vi "FindFacesGrabTester_DEPRECATED.vi"() -> ()   [LabVIEW 2017]
uses:
  Camera_IMAQdx_class/Camera_IMAQdx.lvclass
  Camera_IMAQdx_class/typedefs/Configuration--Cluster.ctl
  ImageFacialDetection_class/ImageFacialDetection.lvclass
  <userlib>/_OpenG.lib/comparison/comparison.llb/Boolean Changed__ogtk.vi
  <vilib>/vision/Image Controls.llb/IMAQ Image.ctl
  <vilib>/userdefined/High Color/IMAQdx.ctl
panel:
  in  "Find Faces":bool
  in  "Refresh List":bool
  in  "Snap":bool
  in  "Start Stop Grab":bool
  in  "Connect to Camera":bool
  in  "Cameras":u16(ring) items=["VMware Virtual USB Video Device "]
  out "Image":T1(plugin-control)
  in  "OK":bool
  out "Frame Number:":u32
  out "Connected":bool
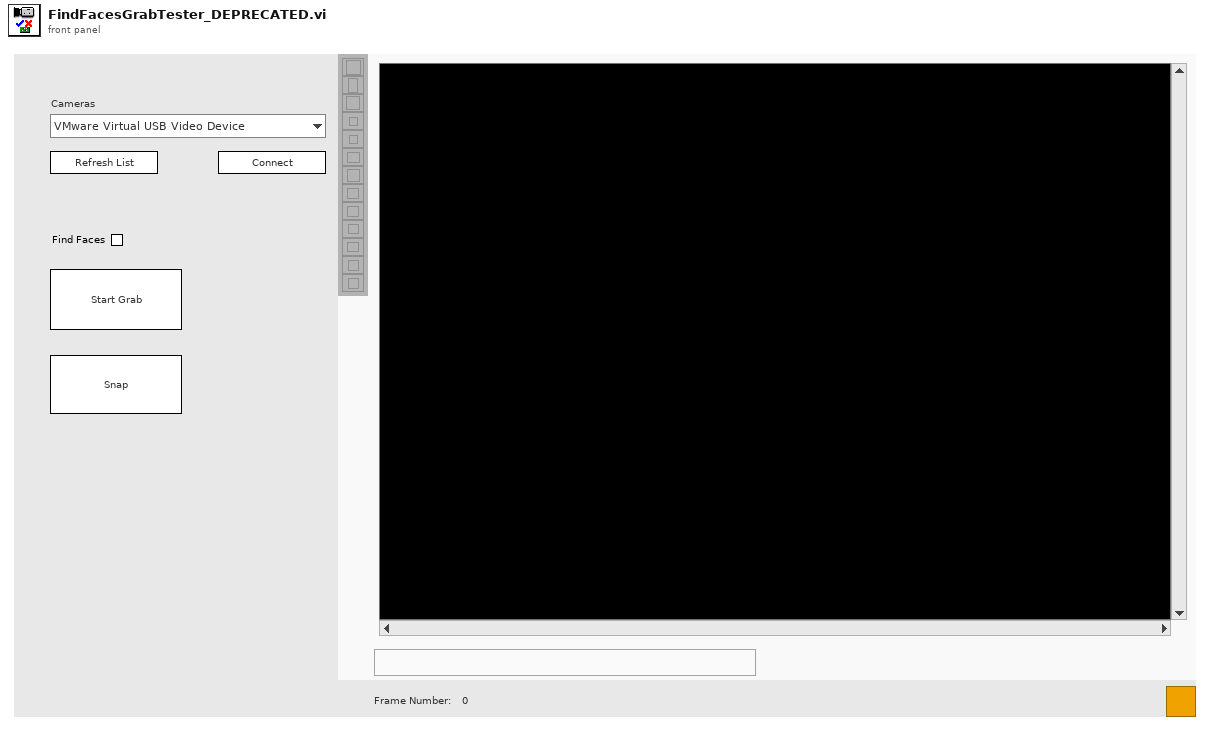
[diagram p1: front panel]
types:
  T1 = typedef "IMAQ Image.ctl" = refnum<image>
  T2 = typedef "Camera_IMAQdx.lvclass/Configuration--Cluster.ctl" = cluster{"Camera Interface Name":string, "Number of Buffers":u32, "Image Name":string, "Image Type":T3}
  T3 = typedef "Image Type" = u32
  T4 = enum32{"invalid app kind", "Development System", "Run Time System", "Student Edition", "Embedded LabVIEW", "Evaluation", "Custom"}
  T5 = enum8{"Enabled", "Disabled", "Disabled and Grayed Out"}
  T6 = enum32{"Invalid", "Standard", "Closed", "Hidden", "Minimized", "Maximized"}
  T7 = cluster{"Core":cluster{"Current VI Reference":refnum<vi>, "Close Panel on Exit?":bool}, "Camera.IMAQdx":refnum<class "Camera_IMAQdx.lvclass">, "All Camera Interfaces":string[], "Connected":bool, "Grabbing":bool, "Find Faces?":bool, "Facial Detection Initialized":bool, "FacialDetection":refnum<class "ImageFacialDetection.lvclass">, "Image":T1, "Face Found":refnum<user-event>, "Frame Complete Event":refnum<event-registration>, "Frame Number":u32}
  T8 = cluster{"Event Registration Refnum":refnum<event-registration>, "Frame Complete Event":refnum<event-registration>}
  T9 = cluster{"Current VI Reference":refnum<vi>, "Close Panel on Exit?":bool}
  T10 = cluster{"Type":u32, "Version":u32, "Flags":u32, "SerialNumberHigh":u32, "SerialNumberLow":u32, "BusType":u32, "InterfaceName":string, "VendorName":string, "ModelName":string, "CameraFileName":string, "CameraAttributeURL":string}[]
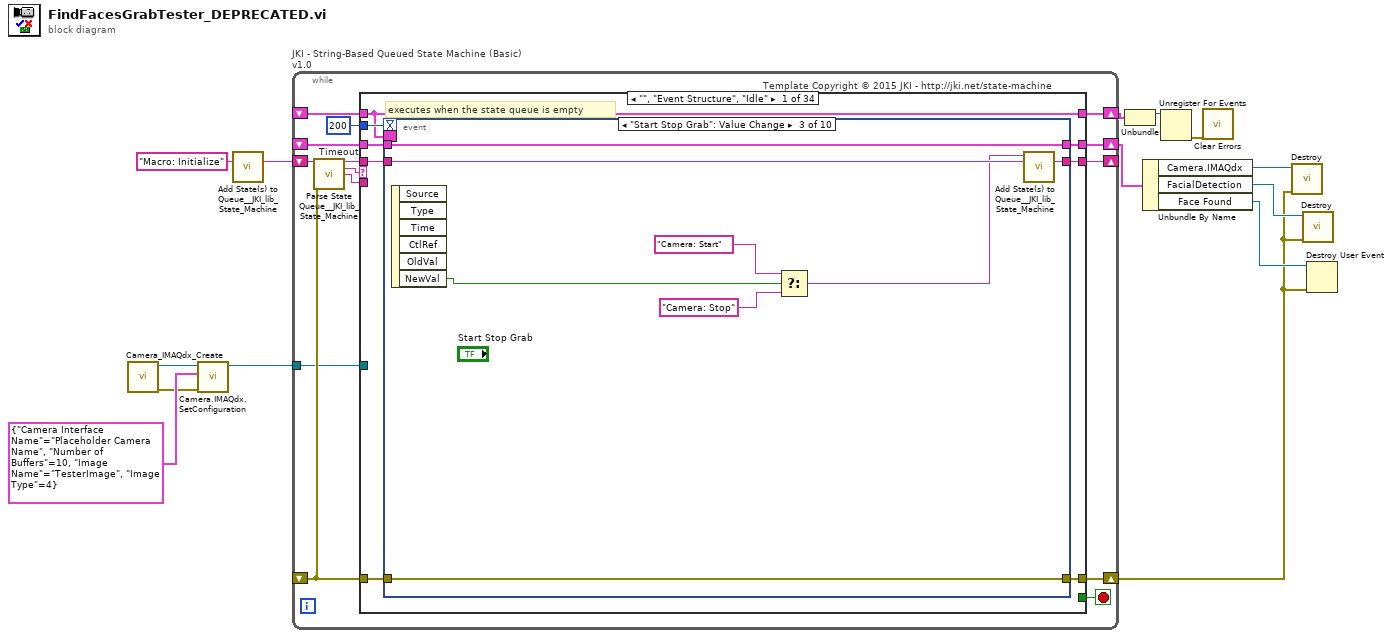
[diagram p0: block diagram]
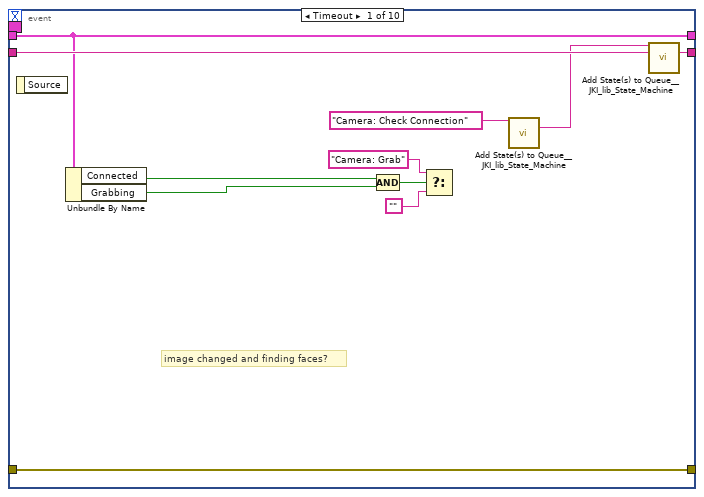
[diagram p2: hidden frame]
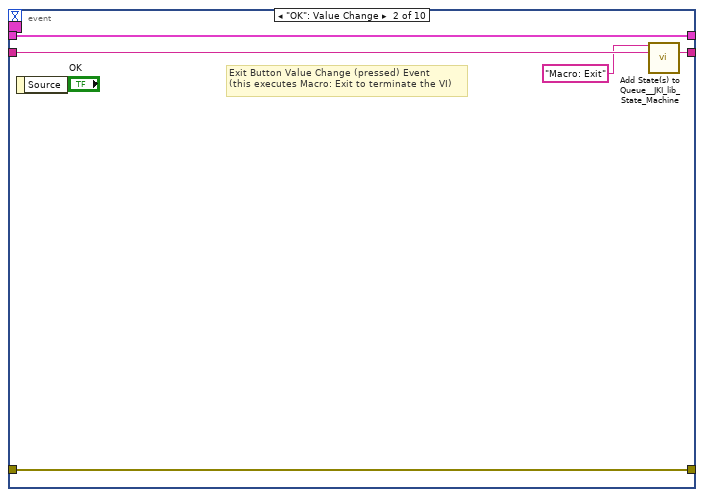
[diagram p3: hidden frame]
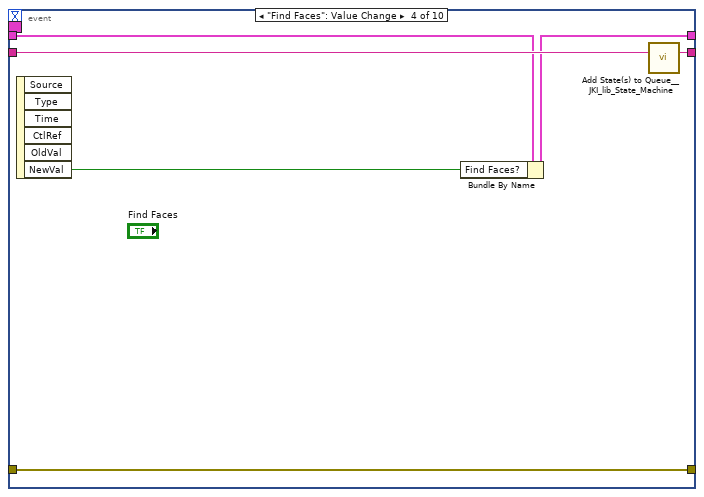
[diagram p4: hidden frame]
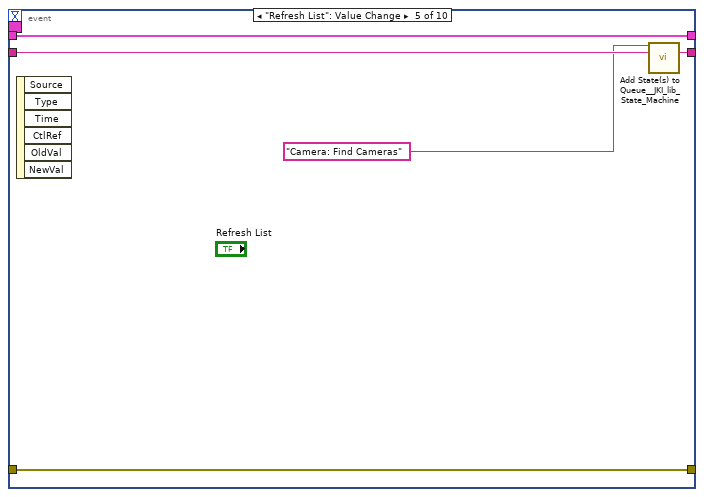
[diagram p5: hidden frame]
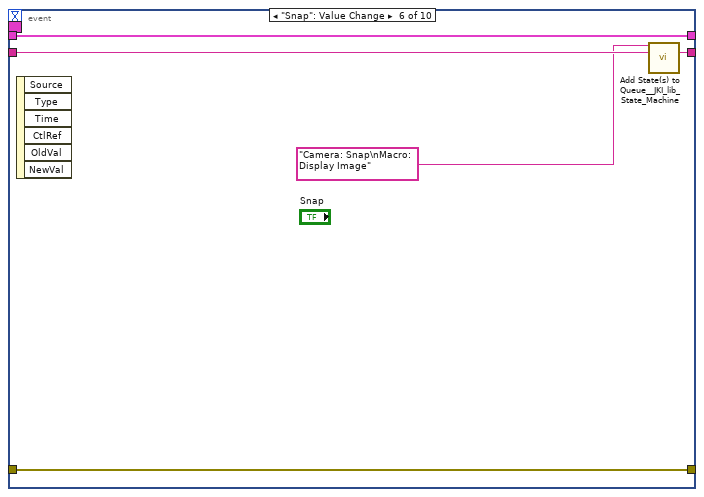
[diagram p6: hidden frame]
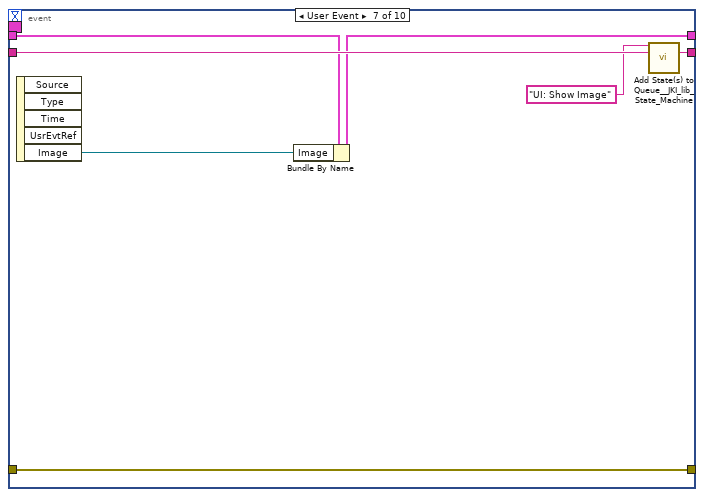
[diagram p7: hidden frame]
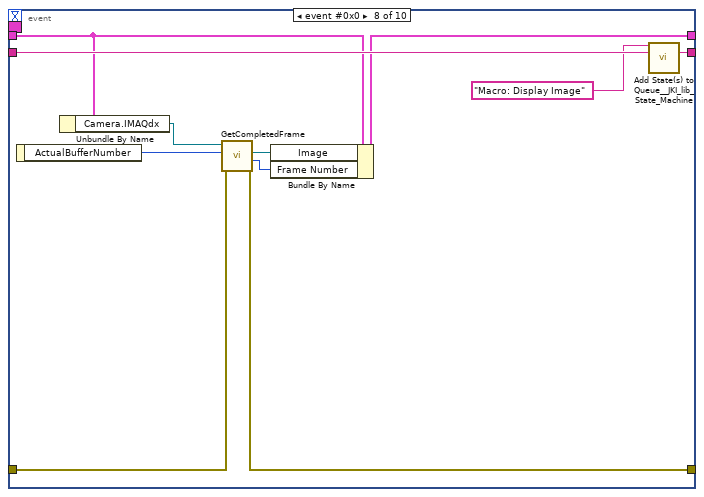
[diagram p8: hidden frame]
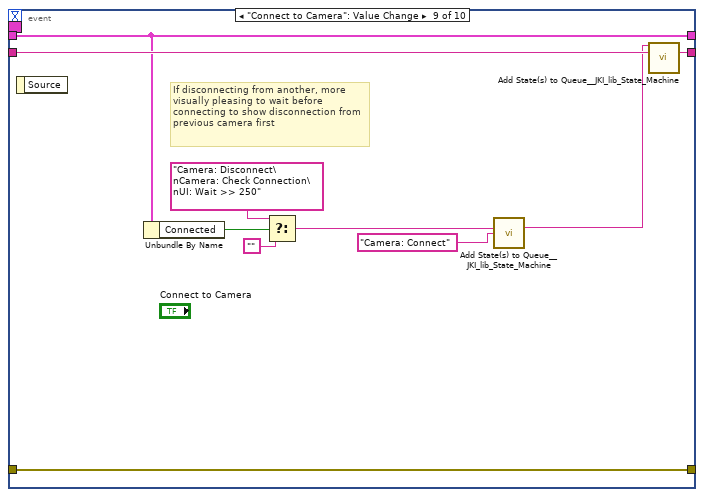
[diagram p9: hidden frame]
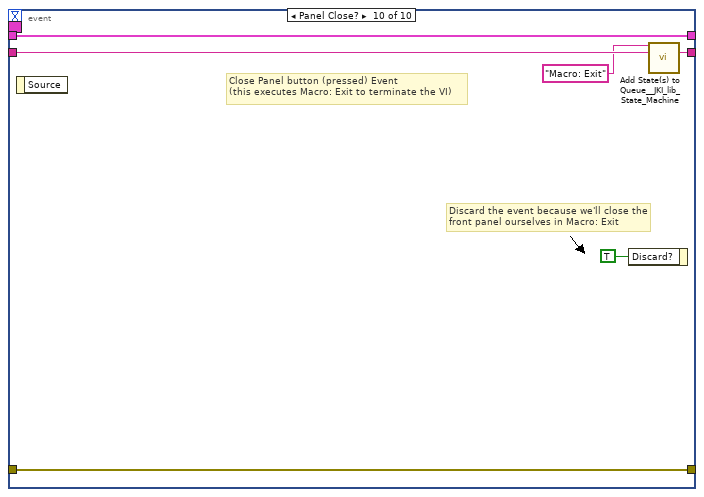
[diagram p10: hidden frame]
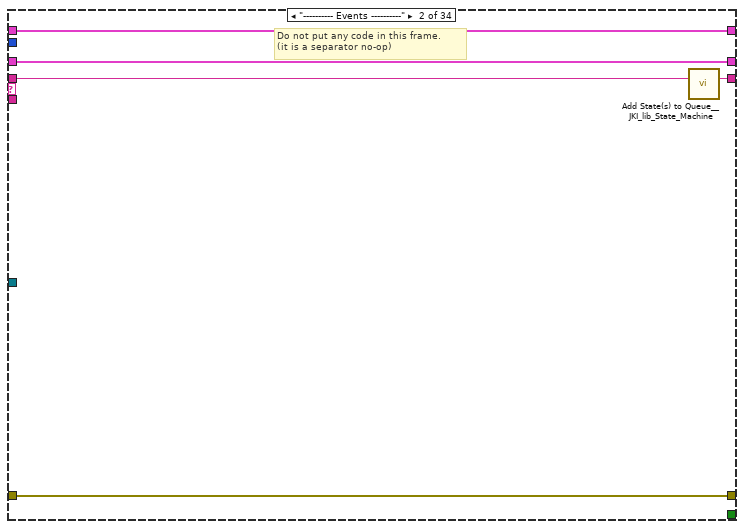
[diagram p11: hidden frame]
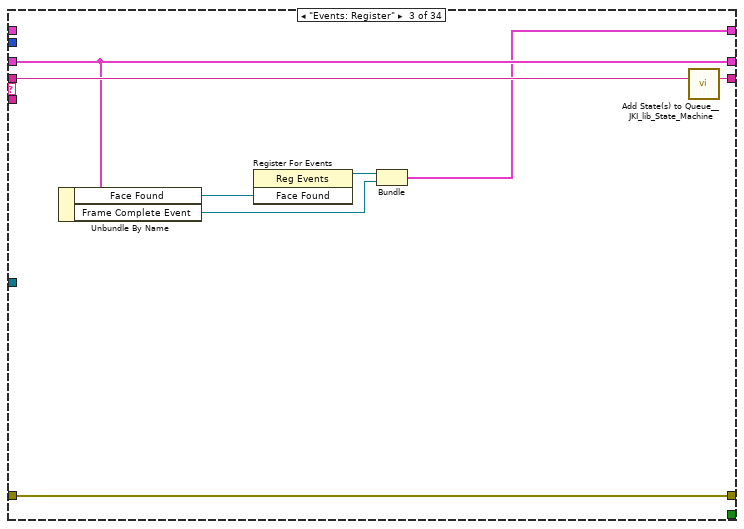
[diagram p12: hidden frame]
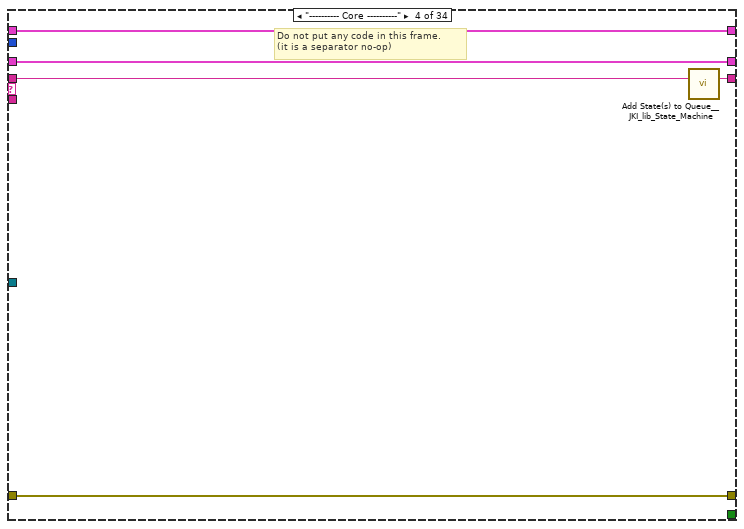
[diagram p13: hidden frame]
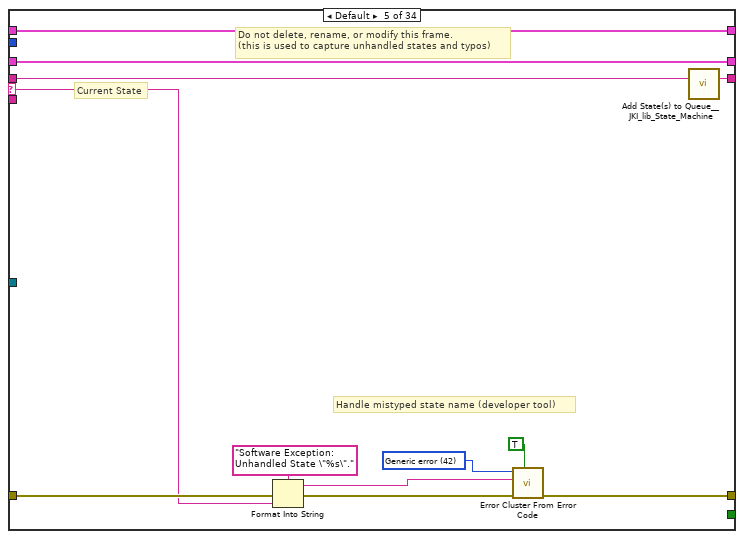
[diagram p14: hidden frame]
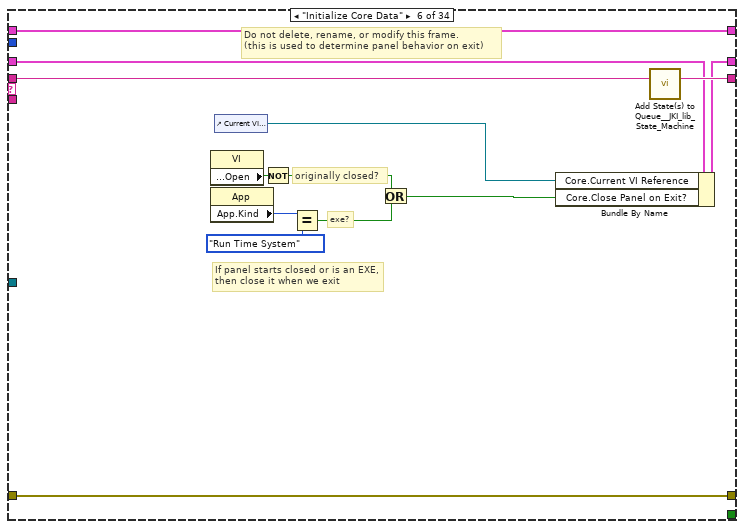
[diagram p15: hidden frame]
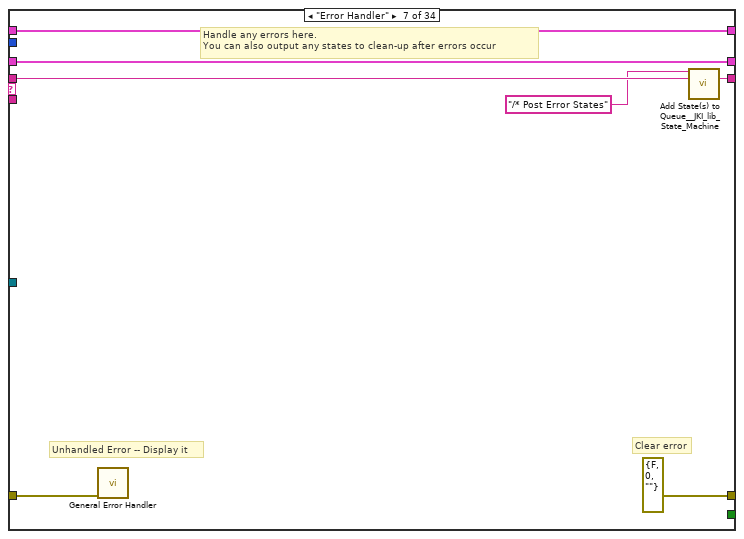
[diagram p16: hidden frame]
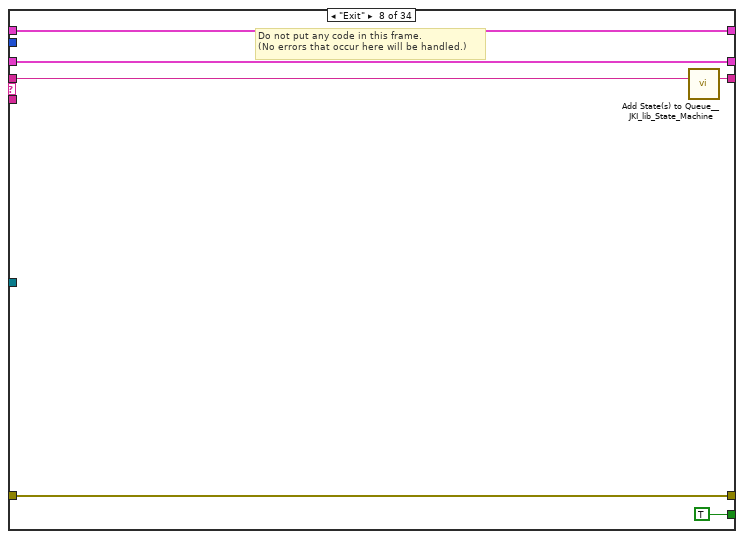
[diagram p17: hidden frame]
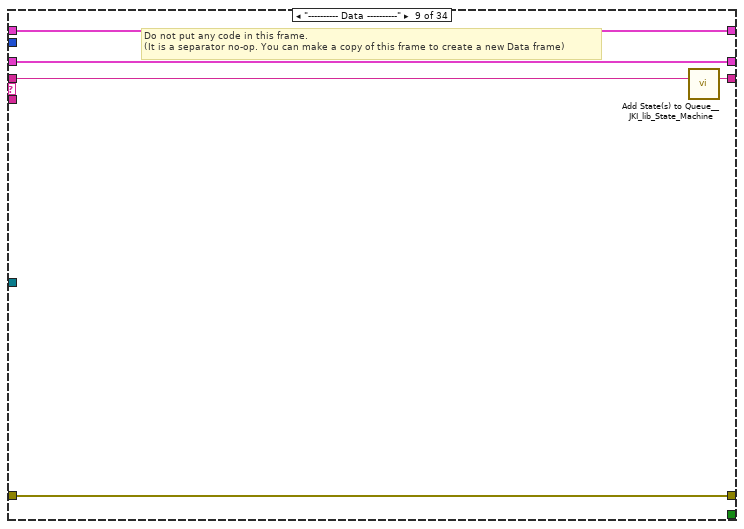
[diagram p18: hidden frame]
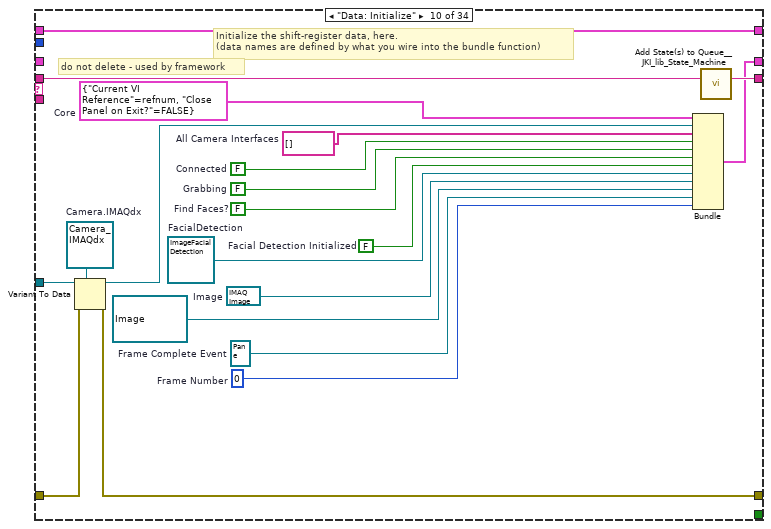
[diagram p19: hidden frame]
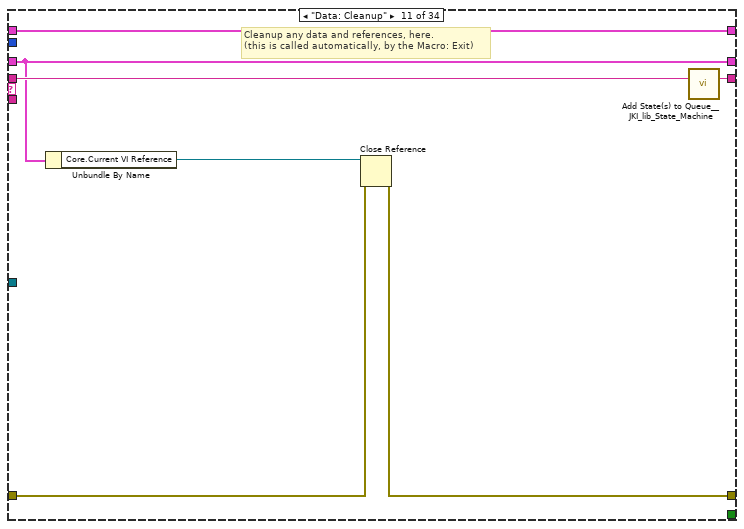
[diagram p20: hidden frame]
diagram:
  n1 = call "Camera_IMAQdx_Create.vi"() -> ("error out"=w7:errorcluster, "reference out"=w12:refnum<class "Camera_IMAQdx.lvclass">)  [unwired: 10 in]
  n2 = call "Camera.IMAQdx.SetConfiguration.vi"("error in (no error)"=w7, "Configuration"=T2 {"Camera Interface Name"="Placeholder Camera Name", "Number of Buffers"=10, "Image Name"="TesterImage", "Image Type"=4}, "reference in"=w12) -> ("reference out"=w9:refnum<class "Camera_IMAQdx.lvclass">)  [unwired: 7 in, 1 out]
  n3 = call <vilib>:"Add State(s) to Queue__JKI_lib_State_Machine.vi"("State(s) in (\"\")"="Macro: Initialize") -> ("States Out"=w14:string)  [unwired: 14 in]
  n4 = while "JKI - String-Based Queued State Machine (Basic) v1.0" {
    shift-right: [w21] -> w11
    shift-left: _ -> [w20]
    shift-right: [w24] -> w4
    shift-left: _ -> [w18]
    shift-right: [w23] -> _
    shift-left: w14 -> [w25]
    tunnel: w9 -> [w17]
    shift-right: [w16] -> w2
    shift-left: _ -> [w15]
    stop <- w22 stop-if-true
    w19 = 200  # Timeout
    # "Template Copyright © 2015 JKI - http://jki.net/state-machine"
    n5 = call <vilib>:"Parse State Queue__JKI_lib_State_Machine.vi"("State Queue"=w25, "Error In (no error)"=w18) -> ("Remaining States"=w27:string, "Current State"=w28:string, "Arguments"=w26:string)  [unwired: 11 in]
    n6 = case shown="\"\", \"Event Structure\", \"Idle\"" w28 {
      selector: w28 -> [_ _ _ _ w130 _ _ _ _ _ _ _ _ _ _ _ _ _ _ _ _ _ _ _ _ _ _ _ _ _ _ _ _ _]
      tunnel: w27 -> [w36 w115 w123 w128 w134 w153 w160 w166 w171 w191 w198 w203 w210 w226 w236 w242 w249 w261 w288 w297 w303 w323 w328 w340 w350 w361 w371 w381 w394 w406 w415 w427 w445 w452]
      tunnel: w26 -> [_ _ _ _ _ _ _ _ _ _ _ _ _ _ w232 _ w244 w255 _ _ _ _ _ _ _ _ _ _ _ _ _ _ _ _]
      tunnel: w20 -> [w34 w112 w120 w125 w132 w144 w157 w164 w168 _ w193 w200 w206 w224 w234 w240 w247 w257 w285 w293 w300 w320 w325 w334 w341 w358 w365 w375 w389 w399 w410 w419 w443 w450]
      tunnel: [w33 w113 w121 w126 w136 w150 errorcluster {"status"=FALSE, "code"=0, "source"=""} ("error out") w163 w169 w180 w194 w201 w208 w216 w233 w239 w245 w258 w286 w295 w301 w321 w326 w331 w342 w359 w367 w377 w390 w402 w411 w422 w435 w447] -> w24
      tunnel: w18 -> [w32 w113 w121 w126 w135 w150 w156 w163 w169 w183 w195 w201 w208 w219 w229 w239 w246 w259 w286 w295 w301 w321 w326 w337 w343 w359 w368 w378 w391 w403 w412 w421 w437 w448]
      tunnel: [w35 w114 w122 w127 w133 w152 w159 w165 w170 w190 w197 w202 w209 w225 w235 w241 w248 w260 w287 w296 w302 w322 w327 w339 w349 w360 w370 w380 w393 w405 w414 w426 w444 w451] -> w23
      tunnel: [_ _ _ _ _ _ _ TRUE _ _ _ _ _ _ _ _ _ _ _ _ _ _ _ _ _ _ _ _ _ _ _ _ _ _] -> w22
      tunnel: [w31 w112 w120 w125 w132 w151 w157 w164 w168 w189 w193 w200 w206 w224 w234 w240 w247 w257 w285 w293 w300 w320 w325 w335 w341 w358 w364 w374 w388 w398 w409 w418 w443 w450] -> w21
      tunnel: w19 -> [w30 _ _ _ _ _ _ _ _ _ _ _ _ _ _ _ _ _ _ _ _ _ _ _ _ _ _ _ _ _ _ _ _ _]
      tunnel: w17 -> [_ _ _ _ _ _ _ _ _ w187 _ _ _ _ _ _ _ _ _ _ _ _ _ _ _ _ _ _ _ _ _ _ _ _]
      tunnel: [w29 w111 w116 w124 w129 w141 w154 w161 w167 w176 w192 w199 w207 w211 w227 w237 w243 w254 w284 w294 w298 w304 w324 w330 w348 w357 w366 w376 w382 w396 w407 w416 w434 w446] -> w16
      tunnel: w15 -> [w29 w111 _ w124 w129 w141 w154 w161 w167 w176 w192 w199 w207 w211 w227 w237 w243 w254 w284 w294 w298 w304 w324 w330 w348 w357 w366 w376 w382 w397 w407 w416 w434 w446]
      frame "", "Event Structure", "Idle" {
        # "executes when the state queue is empty"
        n7 = event shown="[2] \"Start Stop Grab\": Value Change" {
          selector: w29 -> [_ _ _ _ _ _ _ _ _ _]
          dyn-events: _ -> [_ _ _ _ _ _ _ _ _ _]
          timeout: w30 -> [_ _ _ _ _ _ _ _ _ _]
          tunnel: w36 -> [w47 w52 w60 w66 w71 w76 w83 w94 w104 w110]
          tunnel: [w46 w51 w59 w65 w70 w75 w82 w93 w103 w109] -> w35
          tunnel: w34 -> [w44 w49 w57 w63 w68 w73 w80 w89 w101 w107]
          tunnel: [w45 w50 w58 w64 w69 w74 w81 w85 w102 w108] -> w33
          tunnel: w32 -> [w45 w50 w58 w64 w69 w74 w81 w86 w102 w108]
          tunnel: [w44 w49 w57 w62 w68 w73 w79 w92 w101 w107] -> w31
          event Timeout {
            # "image changed and finding faces?"
            n8 = event-data() -> ()  [unwired: 1 in, 1 out]
            n9 = Unbundle By Name(w44) -> ("Connected"=w43:bool, "Grabbing"=w42:bool)
            n10 = Compound Arithmetic op=AND(w43, w42) -> (w41:bool)
            n11 = Select(t="Camera: Grab", s=w41, f="") -> ()  [unwired: 1 out]
            n12 = call <vilib>:"Add State(s) to Queue__JKI_lib_State_Machine.vi"("State(s) in Front (\"\")"="Camera: Check Connection") -> ("States Out"=w37:string)  [unwired: 14 in]
            n13 = call <vilib>:"Add State(s) to Queue__JKI_lib_State_Machine.vi"("State(s) in Front (\"\")"=w37, "State(s) in (\"\")"=w47) -> ("States Out"=w46:string)  [unwired: 13 in]
          }
          event "OK": Value Change {
            # "Exit Button Value Change (pressed) Event\n(this executes Macro: Exit to terminate the VI)"
            n14 = event-data() -> ()  [unwired: 1 in, 1 out]
            n15 = call <vilib>:"Add State(s) to Queue__JKI_lib_State_Machine.vi"("State(s) in Front (\"\")"="Macro: Exit", "State(s) in (\"\")"=w52) -> ("States Out"=w51:string)  [unwired: 13 in]
          }
          event "Start Stop Grab": Value Change {
            n16 = event-data() -> ("NewVal"=w54:bool)  [unwired: 1 in, 5 out]
            n17 = Select(t="Camera: Start", s=w54, f="Camera: Stop") -> (s? t:f=w53:string)
            n18 = call <vilib>:"Add State(s) to Queue__JKI_lib_State_Machine.vi"("State(s) in Front (\"\")"=w53, "State(s) in (\"\")"=w60) -> ("States Out"=w59:string)  [unwired: 13 in]
          }
          event "Find Faces": Value Change {
            n19 = event-data() -> ("NewVal"=w61:bool)  [unwired: 1 in, 5 out]
            n20 = Bundle By Name(cluster=w63, "Find Faces?"=w61) -> (w62:T7)
            n21 = call <vilib>:"Add State(s) to Queue__JKI_lib_State_Machine.vi"("State(s) in (\"\")"=w66) -> ("States Out"=w65:string)  [unwired: 14 in]
          }
          event "Refresh List": Value Change {
            n22 = event-data() -> ()  [unwired: 1 in, 6 out]
            n23 = call <vilib>:"Add State(s) to Queue__JKI_lib_State_Machine.vi"("State(s) in Front (\"\")"="Camera: Find Cameras", "State(s) in (\"\")"=w71) -> ("States Out"=w70:string)  [unwired: 13 in]
          }
          event "Snap": Value Change {
            n24 = event-data() -> ()  [unwired: 1 in, 6 out]
            n25 = call <vilib>:"Add State(s) to Queue__JKI_lib_State_Machine.vi"("State(s) in Front (\"\")"="Camera: Snap\nMacro: Display Image", "State(s) in (\"\")"=w76) -> ("States Out"=w75:string)  [unwired: 13 in]
          }
          event User Event {
            n26 = event-data() -> ("Image"=w78:T1)  [unwired: 1 in, 4 out]
            n27 = Bundle By Name(cluster=w80, "Image"=w78) -> (w79:T7)
            n28 = call <vilib>:"Add State(s) to Queue__JKI_lib_State_Machine.vi"("State(s) in Front (\"\")"="UI: Show Image", "State(s) in (\"\")"=w83) -> ("States Out"=w82:string)  [unwired: 13 in]
          }
          event event #0x0 {
            n29 = event-data() -> ("ActualBufferNumber"=w90:u32)  [unwired: 1 in]
            n30 = Unbundle By Name(w89) -> ("Camera.IMAQdx"=w88:refnum<class "Camera_IMAQdx.lvclass">)
            n31 = call-dynamic "GetCompletedFrame.vi"("error in (no error)"=w86, "ActualBufferNumber"=w90, "reference in"=w88) -> ("error out"=w85:errorcluster, "Frame Number"=w84:u32, "Image Out"=w87:T1)  [unwired: 5 in, 1 out]
            n32 = Bundle By Name(cluster=w89, "Image"=w87, "Frame Number"=w84) -> (w92:T7)
            n33 = call <vilib>:"Add State(s) to Queue__JKI_lib_State_Machine.vi"("State(s) in Front (\"\")"="Macro: Display Image", "State(s) in (\"\")"=w94) -> ("States Out"=w93:string)  [unwired: 13 in]
          }
          event "Connect to Camera": Value Change {
            # "If disconnecting from another, more visually pleasing to wait before connecting to show disconnection from previous camera first"
            n34 = event-data() -> ()  [unwired: 1 in, 1 out]
            n35 = Unbundle By Name(w101) -> ("Connected"=w100:bool)
            n36 = Select(t="Camera: Disconnect\nCamera: Check Connection\nUI: Wait >> 250", s=w100, f="") -> (s? t:f=w97:string)
            n37 = call <vilib>:"Add State(s) to Queue__JKI_lib_State_Machine.vi"("State(s) in (\"\")"=w97, "State(s) at Back (\"\")"="Camera: Connect") -> ("States Out"=w95:string)  [unwired: 13 in]
            n38 = call <vilib>:"Add State(s) to Queue__JKI_lib_State_Machine.vi"("State(s) in Front (\"\")"=w95, "State(s) in (\"\")"=w104) -> ("States Out"=w103:string)  [unwired: 13 in]
          }
          event Panel Close? {
            # "Discard the event because we'll close the front panel ourselves in Macro: Exit"
            # "Close Panel button (pressed) Event\n(this executes Macro: Exit to terminate the VI)"
            n39 = event-data() -> ()  [unwired: 1 in, 1 out]
            n40 = event-data("Discard?"=TRUE) -> ()  [unwired: 1 in, 1 out]
            n41 = call <vilib>:"Add State(s) to Queue__JKI_lib_State_Machine.vi"("State(s) in Front (\"\")"="Macro: Exit", "State(s) in (\"\")"=w110) -> ("States Out"=w109:string)  [unwired: 13 in]
          }
        }
      }
      frame "---------- Events ----------" {
        # "Do not put any code in this frame.\n(it is a separator no-op)"
        n42 = call <vilib>:"Add State(s) to Queue__JKI_lib_State_Machine.vi"("State(s) in (\"\")"=w115) -> ("States Out"=w114:string)  [unwired: 14 in]
      }
      frame "Events: Register" {
        n43 = Unbundle By Name(w120) -> ("Face Found"=w119:refnum<user-event>, "Frame Complete Event"=w117:refnum<event-registration>)
        n44 = register-events(w119) -> (reference out=w118:refnum<event-registration>)  [unwired: 2 in, 1 out]
        n45 = Bundle("Event Registration Refnum"=w118, "Frame Complete Event"=w117) -> (w116:T8)  [unwired: 1 in]
        n46 = call <vilib>:"Add State(s) to Queue__JKI_lib_State_Machine.vi"("State(s) in (\"\")"=w123) -> ("States Out"=w122:string)  [unwired: 14 in]
      }
      frame "---------- Core ----------" {
        # "Do not put any code in this frame.\n(it is a separator no-op)"
        n47 = call <vilib>:"Add State(s) to Queue__JKI_lib_State_Machine.vi"("State(s) in (\"\")"=w128) -> ("States Out"=w127:string)  [unwired: 14 in]
      }
      frame Default {
        w139 = 42 items=["No error", "Argument error", "Memory is full", "Out of zone", "End of file", "File already open", "Generic file I/O error", "File not found", "File permission error", "Disk is full", "Duplicate path", "Too many files open", "System feature not enabled", "Resource file not found", "Cannot add resource", "Resource not found", "Image not found", "Image memory error", "Pen does not exist", "Config type invalid", "Config token not found", "Config parse error", "Config memory error", "Bad external code format", "Bad external code offset", "External code not present", "Null window", "Destroy window error", "Null menu", "Print aborted", "Bad print record", "Print driver error", "Windows error during printing", "Memory error during printing", "Print dialog error", "Generic print error", "Invalid device refnum", "Device not found", "Device parameter error", "Device unit error", "Cannot open device", "Device call aborted", "Generic error", "Cancelled by user", "Object ID too low", "Object ID too high", "Object not in heap", "Unknown heap", "Unknown object (invalid DefProc)", "Unknown object (DefProc not in table)", "Message out of range", "Invalid (null) method", "Unknown message", "Manager call not supported", "Bad address", "Network operation in progress", "Network operation timed out", "Connection is busy", "Network attribute not supported", "Network error", "Address in use", "System out of memory", "Connection aborted", "Connection refused", "Not connected", "Already connected", "Connection closed", "Initialization error (interapplication manager)", "Bad occurrence", "Wait on unbound occurrence handler", "Occurrence queue overflow", "Datalog type conflict", "Unused", "Unrecognized type (interapplication manager)", "Memory corrupt", "Failed to make temporary DLL", "Old CIN version", "Drag socket not found", "Failed to load drop-object", "Failed to register OLE object", "Failed to release OLE object", "Format specifier type mismatch", "Unknown format specifier", "Too few format specifiers", "Too many format specifiers", "Scan failed", "Newer CIN version", "Error converting to variant", "Runtime menu error", "Password tampered", "Variant attribute not found", "Incompatible variant data type", "Event data is not available", "Event Store is not present", "Occurrence is not found", "Event Queue is not created", "Event info is not available", "Refnum passed is NULL", "Error retrieving Class GUID", "Error retrieving CoClass GUID", "Error retrieving TypeLib GUID.", "Bad built application magic bytes.", "Specific driver is different from the specific driver associated with the Logical Name.", "There is no session opened to the class driver.", "Max Error", "MAX - Error with config objects", "MAX - Error loading configuration", "MAX - Group not supported"]
        # "Current State"
        # "Do not delete, rename, or modify this frame.\n(this is used to capture unhandled states and typos)"
        # "Handle mistyped state name (developer tool)"
        n48 = Format Into String(format string="Software Exception: Unhandled State \"%s\"." ("message"), error in=w135, w130) -> (resulting string=w138:string, error out=w137:errorcluster)  [unwired: 1 in]
        n49 = call <vilib>:"Error Cluster From Error Code.vi"("show call chain? (False)"=TRUE, "error in (no error)"=w137, "error message (\"\")"=w138, "error code (0)"=w139) -> ("error out"=w136:errorcluster)  [unwired: 5 in]
        n50 = call <vilib>:"Add State(s) to Queue__JKI_lib_State_Machine.vi"("State(s) in (\"\")"=w134) -> ("States Out"=w133:string)  [unwired: 14 in]
      }
      frame "Initialize Core Data" {
        # "Do not delete, rename, or modify this frame.\n(this is used to determine panel behavior on exit)"
        # "originally closed?"
        # "exe?"
        # "If panel starts closed or is an EXE, then close it when we exit"
        n51 = property class="VI"() -> ("Front Panel.Open"=w149:bool)  [unwired: 2 in, 2 out]
        n52 = property class="App"() -> ("App.Kind"=w148:T4)  [unwired: 2 in, 2 out]
        n53 = control-ref of="Current VI Reference"() -> (w142:refnum<vi>)
        n54 = Not(x=w149) -> (.not. x?=w146:bool)
        n55 = Equal?(x=w148, y=T4."Run Time System" ("Application:Kind")) -> (x = y?=w145:bool)
        n56 = Or(x=w146, y=w145) -> (x .or. y?=w143:bool)
        n57 = Bundle By Name(cluster=w144, "Core.Current VI Reference"=w142, "Core.Close Panel on Exit?"=w143) -> (w151:T7)
        n58 = call <vilib>:"Add State(s) to Queue__JKI_lib_State_Machine.vi"("State(s) in (\"\")"=w153) -> ("States Out"=w152:string)  [unwired: 14 in]
      }
      frame "Error Handler" {
        # "Unhandled Error -- Display it"
        # "Handle any errors here.\nYou can also output any states to clean-up after errors occur"
        # "Clear error"
        n59 = call <vilib>:"General Error Handler.vi"("error in (no error)"=w156) -> ()  [unwired: 10 in, 5 out]
        n60 = call <vilib>:"Add State(s) to Queue__JKI_lib_State_Machine.vi"("State(s) in Front (\"\")"="/* Post Error States", "State(s) in (\"\")"=w160) -> ("States Out"=w159:string)  [unwired: 13 in]
      }
      frame "Exit" {
        # "Do not put any code in this frame.\n(No errors that occur here will be handled.)"
        n61 = call <vilib>:"Add State(s) to Queue__JKI_lib_State_Machine.vi"("State(s) in (\"\")"=w166) -> ("States Out"=w165:string)  [unwired: 14 in]
      }
      frame "---------- Data ----------" {
        # "Do not put any code in this frame.\n(It is a separator no-op. You can make a copy of this frame to create a new Data frame)"
        n62 = call <vilib>:"Add State(s) to Queue__JKI_lib_State_Machine.vi"("State(s) in (\"\")"=w171) -> ("States Out"=w170:string)  [unwired: 14 in]
      }
      frame "Data: Initialize" {
        w172 = u32 0  # Frame Number
        w173 = refnum<event-registration> refnum  # Frame Complete Event
        w175 = T1 refnum  # Image
        w177 = FALSE  # Facial Detection Initialized
        w179 = FALSE  # Find Faces?
        w178 = refnum<class "ImageFacialDetection.lvclass"> refnum  # FacialDetection
        w181 = FALSE  # Grabbing
        w182 = FALSE  # Connected
        w185 = refnum<class "Camera_IMAQdx.lvclass"> refnum  # Camera.IMAQdx
        w186 = string[] []  # All Camera Interfaces
        w188 = T9 {"Current VI Reference"=refnum, "Close Panel on Exit?"=FALSE}  # Core
        # "do not delete - used by framework"
        # "Initialize the shift-register data, here.\n(data names are defined by what you wire into the bundle function)"
        n63 = Variant To Data(error in=w183, type=w185, Variant=w187) -> (data=w184:refnum<class "Camera_IMAQdx.lvclass">, error out=w180:errorcluster)
        n64 = Bundle("Core"=w188, "Camera.IMAQdx"=w184, "All Camera Interfaces"=w186, "Connected"=w182, "Grabbing"=w181, "Find Faces?"=w179, "Facial Detection Initialized"=w177, "FacialDetection"=w178, "Image"=w175, "Face Found"=refnum<user-event> refnum, "Frame Complete Event"=w173, "Frame Number"=w172) -> (w189:T7)  [unwired: 1 in]
        n65 = call <vilib>:"Add State(s) to Queue__JKI_lib_State_Machine.vi"("State(s) in (\"\")"=w191) -> ("States Out"=w190:string)  [unwired: 14 in]
      }
      frame "Data: Cleanup" {
        # "Cleanup any data and references, here.\n(this is called automatically, by the Macro: Exit)"
        n66 = Unbundle By Name(w193) -> ("Core.Current VI Reference"=w196:refnum<vi>)
        n67 = Close Reference(reference=w196, error in (no error)=w195) -> (error out=w194:errorcluster)
        n68 = call <vilib>:"Add State(s) to Queue__JKI_lib_State_Machine.vi"("State(s) in (\"\")"=w198) -> ("States Out"=w197:string)  [unwired: 14 in]
      }
      frame "---------- UI ----------" {
        # "Do not put any code in this frame.\n(It is a separator no-op. You can make a copy of this frame to create a new UI frame)"
        n69 = call <vilib>:"Add State(s) to Queue__JKI_lib_State_Machine.vi"("State(s) in (\"\")"=w203) -> ("States Out"=w202:string)  [unwired: 14 in]
      }
      frame "UI: Show Image" {
        n70 = Unbundle By Name(w206) -> ("Image"=→"Image":T1, "Frame Number"=→"Frame Number:":u32)
        n71 = call <vilib>:"Add State(s) to Queue__JKI_lib_State_Machine.vi"("State(s) in (\"\")"=w210) -> ("States Out"=w209:string)  [unwired: 14 in]
      }
      frame "UI: Update Interlock" {
        n72 = Unbundle By Name(w224) -> ("Connected"=w223:bool, "Facial Detection Initialized"=w213:bool)
        n73 = Select(t=T5."Enabled" ("Disabled"), s=w213, f=T5."Disabled and Grayed Out" ("Disabled")) -> (s? t:f=w212:T5)
        n74 = Select(t=T5."Enabled" ("Disabled"), s=w223, f=T5."Disabled and Grayed Out" ("Disabled")) -> (s? t:f=w218:T5)
        n75 = property on="Start Stop Grab" class="Bool (strict)"(error in=w219, "DisabledEnum"=w218) -> (error out=w220:errorcluster)  [unwired: 1 in, 1 out]
        n76 = property on="Snap" class="Bool"(error in=w220, "DisabledEnum"=w218) -> (error out=w217:errorcluster)  [unwired: 1 in, 1 out]
        n77 = property on="Find Faces" class="Bool (strict)"(error in=w217, "DisabledEnum"=w212) -> (error out=w216:errorcluster)  [unwired: 1 in, 1 out]
        n78 = call <vilib>:"Add State(s) to Queue__JKI_lib_State_Machine.vi"("State(s) in (\"\")"=w226) -> ("States Out"=w225:string)  [unwired: 14 in]
      }
      frame "UI: Wait" {
        n79 = Scan From String(format string="%d", input string=w232, error in=w229) -> (error out=w228:errorcluster, output 1=w230:i32)  [unwired: 2 in, 2 out]
        n80 = call <userlib>:"Wait (ms)__ogtk.vi"("error in (no error)"=w228, "milliseconds to wait"=w230) -> ("error out"=w233:errorcluster)  [unwired: 8 in, 1 out]
        n81 = call <vilib>:"Add State(s) to Queue__JKI_lib_State_Machine.vi"("State(s) in (\"\")"=w236) -> ("States Out"=w235:string)  [unwired: 14 in]
      }
      frame "UI: Initialize" {
        w238 = FALSE
        # "Initialize the User Interface, here.\n(this is called automatically, by the Macro: Init)"
        n82 = local write "Find Faces"(w238) -> ()
        n83 = local write "Connected"(w238) -> ()
        n84 = call <vilib>:"Add State(s) to Queue__JKI_lib_State_Machine.vi"("State(s) in (\"\")"=w242) -> ("States Out"=w241:string)  [unwired: 14 in]
      }
      frame "UI: Cursor Set" {
        # "Argument"
        # "Set and Unset Cursor Busy.\n(Usage: \"UI: Cursor Set >> Busy|Idle\")"
        n85 = case shown="\"Idle\", Default" w244 {
          tunnel: w246 -> [w251 w253]
          tunnel: [w250 w252] -> w245
          frame "Idle", Default {
            n86 = call <vilib>:"Unset Busy.vi"("error in (no error)"=w251) -> ("error out"=w250:errorcluster)  [unwired: 10 in]
          }
          frame "Busy" {
            n87 = call <vilib>:"Set Busy.vi"("error in (no error)"=w253) -> ("error out"=w252:errorcluster)  [unwired: 9 in, 1 out]
          }
        }
        n88 = call <vilib>:"Add State(s) to Queue__JKI_lib_State_Machine.vi"("State(s) in (\"\")"=w249) -> ("States Out"=w248:string)  [unwired: 14 in]
      }
      frame "UI: Front Panel State" {
        # "Argument"
        # "Set Front Panel Open or Closed\n(Usage: \"UI: Front Panel State >> Open|Close\")"
        n89 = Unbundle By Name(w257) -> ("Core.Current VI Reference"=w256:refnum<vi>)
        n90 = case shown="\"Open\", Default" w255 {
          tunnel: w259 -> [w265 w278]
          tunnel: [w267 w279] -> w258
          tunnel: w256 -> [w266 w276]
          frame "Open", Default {
            n91 = property class="VI"(reference=w266, error in=w265) -> (reference out=w263:refnum<vi>, error out=w264:errorcluster, "Front Panel.Open"=w262:bool)
            n92 = case shown="False" w262 {
              tunnel: [w270 w273] -> w267
              tunnel: w264 -> [w269 w273]
              tunnel: w263 -> [w268 _]
              frame False {
                n93 = invoke class="VI" method="FP.Open"(reference=w268, error in=w269, "Activate"=TRUE, "State"=T6."Standard") -> (error out=w270:errorcluster)  [unwired: 1 in, 4 out]
              }
              frame True {
              }
            }
          }
          frame "Close" {
            n94 = property class="VI"(reference=w276, error in=w278) -> (reference out=w275:refnum<vi>, error out=w277:errorcluster, "Front Panel.Open"=w274:bool)
            n95 = case shown="True" w274 {
              tunnel: [w280 w283] -> w279
              tunnel: w277 -> [w280 w282]
              tunnel: w275 -> [_ w281]
              frame False {
              }
              frame True {
                n96 = invoke class="VI" method="FP.Close"(reference=w281, error in=w282) -> (error out=w283:errorcluster)  [unwired: 1 in, 2 out]
              }
            }
          }
        }
        n97 = call <vilib>:"Add State(s) to Queue__JKI_lib_State_Machine.vi"("State(s) in (\"\")"=w261) -> ("States Out"=w260:string)  [unwired: 14 in]
      }
      frame "---------- Macro ----------" {
        # "Do not put any code in this frame.\n(It is a separator no-op. You can make a copy of this frame to create a new Macro frame)"
        n98 = call <vilib>:"Add State(s) to Queue__JKI_lib_State_Machine.vi"("State(s) in (\"\")"=w288) -> ("States Out"=w287:string)  [unwired: 14 in]
      }
      frame "Macro: Display Image" {
        # "If finding faces the face found event will return the image to be shown, otherwise show it directly"
        n99 = Unbundle By Name(w293) -> ("Find Faces?"=w292:bool)
        n100 = Select(t="Facial Detection: Find Faces" ("State(s) in Front (\"\")"), s=w292, f="UI: Show Image" ("State(s) in Front (\"\")")) -> (s? t:f=w289:string)
        n101 = call <vilib>:"Add State(s) to Queue__JKI_lib_State_Machine.vi"("State(s) in Front (\"\")"=w289, "State(s) in (\"\")"=w297) -> ("States Out"=w296:string)  [unwired: 13 in]
      }
      frame "Macro: Initialize" {
        w299 = "Data: Initialize\nInitialize Core Data\nUI: Initialize\nUI: Update Interlock\nUI: Cursor Set >> Busy\nCamera: Find Cameras\nFacial Detection: Create\nEvents: Register\nUI: Update Interlock\nUI: Cursor Set >> Idle\nUI: Front Panel State >> Open"  # Data: Initialize Initialize Core Data UI: Initialize UI: Update Interlock UI: Cursor Set >> Busy Camera: Find Cameras Facial Detection: Create Events: Register UI: Update Interlock UI: Cursor Set >> Idle UI: Front Panel State >> Open
        # "Initialization Macro\n(This is called once, when the VI starts)"
        n102 = call <vilib>:"Add State(s) to Queue__JKI_lib_State_Machine.vi"("State(s) in Front (\"\")"=w299, "State(s) in (\"\")"=w303) -> ("States Out"=w302:string)  [unwired: 13 in]
      }
      frame "Macro: Exit" {
        # "Exit Macro\n(This is called once, when the VI exits)"
        n103 = Unbundle By Name(w320) -> ("Grabbing"=w309:bool, "Connected"=w308:bool, "Core.Close Panel on Exit?"=w319:bool)
        n104 = Select(t="Camera: Stop", s=w309, f="") -> (s? t:f=w307:string)
        n105 = Select(t="Camera: Disconnect", s=w308, f="") -> (s? t:f=w306:string)
        n106 = Select(t="UI: Front Panel State >> Close", s=w319, f="") -> (s? t:f=w316:string)
        n107 = call <vilib>:"Add State(s) to Queue__JKI_lib_State_Machine.vi"("State(s) in Front (\"\")"=w307, "State(s) in (\"\")"=w306) -> ("States Out"=w305:string)  [unwired: 13 in]
        n108 = call <vilib>:"Add State(s) to Queue__JKI_lib_State_Machine.vi"("State(s) in Front (\"\")"=w305, "State(s) in (\"\")"=w316, "State(s) at Back (\"\")"="Data: Cleanup\nExit") -> ("States Out"=w314:string)  [unwired: 12 in]
        n109 = call <vilib>:"Add State(s) to Queue__JKI_lib_State_Machine.vi"("State(s) in Front (\"\")"=w314, "State(s) in (\"\")"=w323) -> ("States Out"=w322:string)  [unwired: 13 in]
      }
      frame "---------- Facial Detection ----------" {
        # "Template Separator\n(You can make a copy of, or modify, this frame)"
        n110 = call <vilib>:"Add State(s) to Queue__JKI_lib_State_Machine.vi"("State(s) in (\"\")"=w328) -> ("States Out"=w327:string)  [unwired: 14 in]
      }
      frame "Facial Detection: Create" {
        n111 = call "ImageFacialDetection_Create.vi"("error in (no error)"=w337) -> ("error out"=w332:errorcluster, "reference out"=w338:refnum<class "ImageFacialDetection.lvclass">)  [unwired: 9 in]
        n112 = Create User Event(user event datatype=T1 refnum ("Image"), error in=w332) -> (user event=w329:refnum<user-event>, error out=w331:errorcluster)
        n113 = Bundle By Name(cluster=w334, "FacialDetection"=w338, "Facial Detection Initialized"=TRUE, "Face Found"=w329) -> (w335:T7)
        n114 = call <vilib>:"Add State(s) to Queue__JKI_lib_State_Machine.vi"("State(s) in (\"\")"=w340) -> ("States Out"=w339:string)  [unwired: 14 in]
      }
      frame "Facial Detection: Find Faces" {
        n115 = Unbundle By Name(w341) -> ("FacialDetection"=w347:refnum<class "ImageFacialDetection.lvclass">, "Image"=w346:T1, "Face Found"=w345:refnum<user-event>, "Find Faces?"=w344:bool)
        n116 = case shown="True" w344 {
          tunnel: w347 -> [_ w356]
          tunnel: w346 -> [_ w355]
          tunnel: w345 -> [_ w354]
          tunnel: w343 -> [w351 w353]
          tunnel: [w351 w352] -> w342
          frame False {
          }
          frame True {
            n117 = call "FindFaces_Async.vi"("error in (no error)"=w353, "Face Detected Event"=w354, "image"=w355, "reference in"=w356) -> ("error out"=w352:errorcluster)  [unwired: 7 in]
          }
        }
        n118 = call <vilib>:"Add State(s) to Queue__JKI_lib_State_Machine.vi"("State(s) in (\"\")"=w350) -> ("States Out"=w349:string)  [unwired: 14 in]
      }
      frame "---------- Camera ----------" {
        # "Template Separator\n(You can make a copy of, or modify, this frame)"
        n119 = call <vilib>:"Add State(s) to Queue__JKI_lib_State_Machine.vi"("State(s) in (\"\")"=w361) -> ("States Out"=w360:string)  [unwired: 14 in]
      }
      frame "Camera: Grab" {
        n120 = Unbundle By Name(w365) -> ("Camera.IMAQdx"=w369:refnum<class "Camera_IMAQdx.lvclass">)  [unwired: 2 out]
        n121 = call-dynamic "Grab.vi"("error in (no error)"=w368, "reference in"=w369) -> ("error out"=w367:errorcluster, "Frame Number"=w362:u32, "Image Out"=w363:T1)  [unwired: 6 in, 1 out]
        n122 = Bundle By Name(cluster=w365, "Image"=w363, "Frame Number"=w362) -> (w364:T7)
        n123 = call <vilib>:"Add State(s) to Queue__JKI_lib_State_Machine.vi"("State(s) in (\"\")"=w371) -> ("States Out"=w370:string)  [unwired: 14 in]
      }
      frame "Camera: Snap" {
        n124 = Unbundle By Name(w375) -> ("Camera.IMAQdx"=w379:refnum<class "Camera_IMAQdx.lvclass">)
        n125 = call-dynamic "Snap.vi"("error in (no error)"=w378, "reference in"=w379) -> ("error out"=w377:errorcluster, "Image Out"=w373:T1)  [unwired: 7 in, 1 out]
        n126 = Bundle By Name(cluster=w375, "Image"=w373, "Frame Number"=u32 1 ("Frame Number:")) -> (w374:T7)
        n127 = call <vilib>:"Add State(s) to Queue__JKI_lib_State_Machine.vi"("State(s) in (\"\")"=w381) -> ("States Out"=w380:string)  [unwired: 14 in]
      }
      frame "Camera: Check Connection" {
        n128 = Unbundle By Name(w389) -> ("Camera.IMAQdx"=w392:refnum<class "Camera_IMAQdx.lvclass">)
        n129 = call-dynamic "GetConnected.vi"("error in (no error)"=w391, "reference in"=w392) -> ("error out"=w390:errorcluster, "Connected"=w387:bool)  [unwired: 7 in, 1 out]
        "Connected" <- w387
        n130 = call-poly <userlib>:"Data Changed__ogtk.vi"("Boolean"=w387) -> ("Changed"=w386:bool)
        n131 = Bundle By Name(cluster=w389, "Connected"=w387) -> (w388:T7)
        n132 = Select(t="UI: Update Interlock", s=w386, f="") -> (s? t:f=w383:string)
        n133 = call <vilib>:"Add State(s) to Queue__JKI_lib_State_Machine.vi"("State(s) in Front (\"\")"=w383, "State(s) in (\"\")"=w394) -> ("States Out"=w393:string)  [unwired: 13 in]
      }
      frame "Camera: Start" {
        n134 = Unbundle By Name(w399) -> ("Camera.IMAQdx"=w404:refnum<class "Camera_IMAQdx.lvclass">)
        n135 = call-dynamic "StartAcquisitionWithEvent.vi"("error in (no error)"=w403, "reference in"=w404) -> ("error out"=w402:errorcluster, "Frame Complete Event"=w395:refnum<event-registration>)  [unwired: 7 in, 1 out]
        n136 = Unbundle By Name(w402) -> ("status"=w401:bool)
        n137 = Bundle By Name(cluster=w397, "Frame Complete Event"=w395) -> (w396:T8)
        n138 = Not(x=w401) -> (.not. x?=w400:bool)
        n139 = Bundle By Name(cluster=w399, "Frame Complete Event"=w395, "Grabbing"=w400) -> (w398:T7)
        n140 = call <vilib>:"Add State(s) to Queue__JKI_lib_State_Machine.vi"("State(s) in (\"\")"=w406) -> ("States Out"=w405:string)  [unwired: 14 in]
      }
      frame "Camera: Stop" {
        n141 = Unbundle By Name(w410) -> ("Camera.IMAQdx"=w413:refnum<class "Camera_IMAQdx.lvclass">)
        n142 = call-dynamic "StopAcquisition.vi"("error in (no error)"=w412, "reference in"=w413) -> ("error out"=w411:errorcluster)  [unwired: 8 in, 1 out]
        n143 = Bundle By Name(cluster=w410, "Grabbing"=FALSE) -> (w409:T7)
        n144 = call <vilib>:"Add State(s) to Queue__JKI_lib_State_Machine.vi"("State(s) in (\"\")"=w415) -> ("States Out"=w414:string)  [unwired: 14 in]
      }
      frame "Camera: Find Cameras" {
        n145 = Unbundle By Name(w419) -> ("Camera.IMAQdx"=w425:refnum<class "Camera_IMAQdx.lvclass">)
        n146 = call "FindCameras.vi"("error in (no error)"=w421, "reference in"=w425) -> ("error out"=w420:errorcluster, "Camera Information Array"=w424:T10)  [unwired: 7 in, 1 out]
        n147 = for {
          tunnel: w424 -> [w433] mode=indexing
          tunnel: [w429] -> w423 mode=indexing
          tunnel: [w428] -> w417 mode=indexing
          n148 = Unbundle By Name(w433) -> ("InterfaceName"=w428:string, "VendorName"=w432:string, "ModelName"=w430:string)
          n149 = call <vilib>:"Space Constant.vi"() -> ("String"=w431:string)
          n150 = Concatenate Strings(w432, w431, w430) -> (w429:string)
        }
        n151 = Bundle By Name(cluster=w419, "All Camera Interfaces"=w417) -> (w418:T7)
        n152 = property on="Cameras" class="Ring (strict)"(error in=w420, "Strings []"=w423) -> (error out=w422:errorcluster)  [unwired: 1 in, 1 out]
        n153 = call <vilib>:"Add State(s) to Queue__JKI_lib_State_Machine.vi"("State(s) in (\"\")"=w427) -> ("States Out"=w426:string)  [unwired: 14 in]
      }
      frame "Camera: Connect" {
        n154 = Unbundle By Name(w443) -> ("Camera.IMAQdx"=w442:refnum<class "Camera_IMAQdx.lvclass">, "All Camera Interfaces"=w440:string[])
        n155 = Index Array(array=w440, index="Cameras") -> (element=w438:string)
        n156 = call "SetCameraInterfaceName.vi"("error in (no error)"=w437, "Camera Interface Name"=w438, "reference in"=w442) -> ("error out"=w436:errorcluster, "reference out"=w441:refnum<class "Camera_IMAQdx.lvclass">)  [unwired: 7 in]
        n157 = call-dynamic "Connect.vi"("error in (no error)"=w436, "reference in"=w441) -> ("error out"=w435:errorcluster)  [unwired: 8 in, 1 out]
        n158 = call <vilib>:"Add State(s) to Queue__JKI_lib_State_Machine.vi"("State(s) in (\"\")"=w445) -> ("States Out"=w444:string)  [unwired: 14 in]
      }
      frame "Camera: Disconnect" {
        n159 = Unbundle By Name(w450) -> ("Camera.IMAQdx"=w449:refnum<class "Camera_IMAQdx.lvclass">)
        n160 = call-dynamic "Disconnect.vi"("error in (no error)"=w448, "reference in"=w449) -> ("error out"=w447:errorcluster)  [unwired: 8 in, 1 out]
        n161 = call <vilib>:"Add State(s) to Queue__JKI_lib_State_Machine.vi"("State(s) in (\"\")"=w452) -> ("States Out"=w451:string)  [unwired: 14 in]
      }
    }
  }
  n162 = Unbundle(w2) -> ("Event Registration Refnum"=w1:refnum<event-registration>)  [unwired: 1 out]
  n163 = Unbundle By Name(w11) -> ("Camera.IMAQdx"=w10:refnum<class "Camera_IMAQdx.lvclass">, "FacialDetection"=w6:refnum<class "ImageFacialDetection.lvclass">, "Face Found"=w5:refnum<user-event>)
  n164 = Unregister For Events(event registration refnum=w1) -> (error out=w3:errorcluster)  [unwired: 1 in]
  n165 = call <vilib>:"Clear Errors.vi"("error in (no error)"=w3) -> ()  [unwired: 5 in, 2 out]
  n166 = call-dynamic "Destroy.vi"("error in (no error)"=w4, "reference in"=w10) -> ()  [unwired: 8 in, 2 out]
  n167 = call-dynamic "Destroy.vi"("error in (no error)"=w4, "reference in"=w6) -> ()  [unwired: 8 in, 2 out]
  n168 = Destroy User Event(user event=w5, error in=w4) -> ()  [unwired: 1 out]
